vi "IAmEngine-CreateDVR-ForIAmGLF.vi"(8 "error in (no error)":errorcluster, 9 "IAmGLF Return Notifier":refnum<notifier>, 10 "IAmGLF To Create DVR":refnum<class "IAmGLF.lvclass">, 11 "Engine in":refnum<class "Engine.lvclass">) -> (0 "error out":errorcluster, 3 "Engine out":refnum<class "Engine.lvclass">)   [LabVIEW 2024, in "GLF.lvlib" / "Engine.lvclass"]
doc: "<B>Summary</B>\nCreate DVR for <B>IAmEngine To Create DVR</B>\n\n<B>Details</B>\nThis is really here to reduce coupling between GLF classes. Engine will depend on other classes (Window, View, etc...). But the way I want to use them would require them to depend on Engine too, inducing circular dependency."
uses:
  Engine.lvclass
  Engine.lvclass/Engine.ctl
  Command--enum.ctl
  IAmGLF/IAmGLF.lvclass
  Command-CreateDVR--cluster.ctl
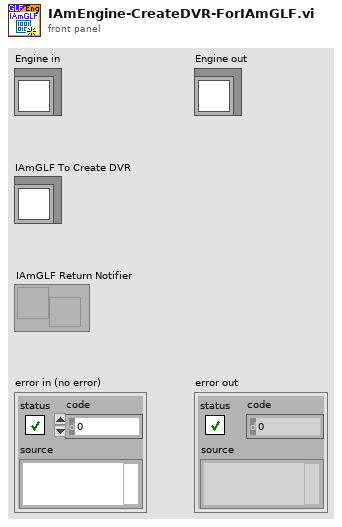
[diagram p1: front panel]
types:
  T1 = typedef "GLF.lvlib/Engine.lvclass/Command-CreateDVR--cluster.ctl" = cluster{"IAmGLF To Create DVR":refnum<class "IAmGLF.lvclass">, "IAmGLF Return Notifier":refnum<notifier>}
  T2 = typedef "GLF.lvlib/Engine.lvclass/Command--enum.ctl" = enum16{"Quit", "Create DVR"}
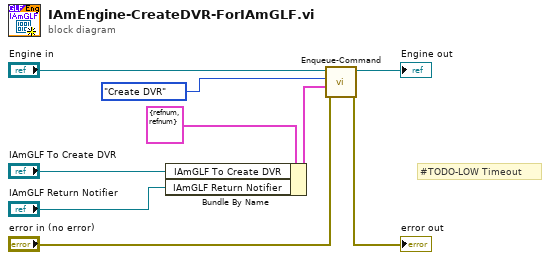
[diagram p0: block diagram]
diagram:
  # "#TODO-LOW Timeout"
  n1 = Bundle By Name(cluster=T1 {"IAmGLF To Create DVR"=refnum, "IAmGLF Return Notifier"=refnum} ("Data"), "IAmGLF To Create DVR"="IAmGLF To Create DVR", "IAmGLF Return Notifier"="IAmGLF Return Notifier") -> (w1:T1)
  n2 = call "Enqueue-Command.vi"("error in (no error)"="error in (no error)", "Cmd Data"=w1, "Cmd"=Command--enum."Create DVR", "Engine in"="Engine in") -> ("error out"=→"error out":errorcluster, "Engine out"=→"Engine out":refnum<class "Engine.lvclass">)  [unwired: 5 in, 1 out]
